vi "Joystick Control.vi"(10 "RobotDriveDevRef":T1={"DevStatus"={"status"=FALSE, "code"=0, "source"=""}, "Motors[]"=[], "Square Inputs"=FALSE, "Max Output"=1.0}) -> ()   [LabVIEW 2019]
uses:
  <vilib>/Rock Robotics/WPI/RobotDrive/WPI_RobotDriveDevRef.ctl
  <vilib>/Rock Robotics/WPI/MotorControl/WPI_MotorControlDeviceRef.ctl
  <vilib>/Rock Robotics/WPI/MotorControl/WPI_MotorControlType.ctl
  <vilib>/Rock Robotics/SystemInterfaces/DIO/FPGA_DIOPWMChannel.ctl
  <vilib>/Rock Robotics/WPI/PWM/WPI_PWMDeadband.ctl
  <vilib>/Rock Robotics/SystemInterfaces/DIO/FPGA_DIOChannel.ctl
  Robot Global Data.vi
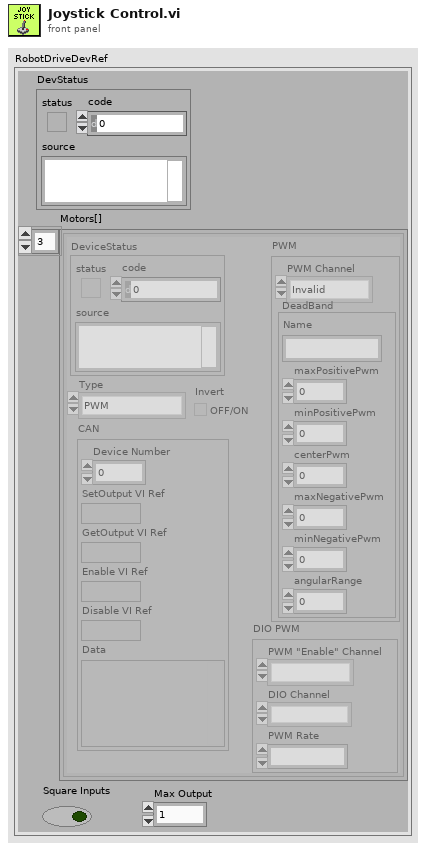
[diagram p1: front panel]
types:
  T1 = typedef "WPI_RobotDriveDevRef.ctl" = cluster{"DevStatus":errorcluster, "Motors[]":T2[], "Square Inputs":bool, "Max Output":dbl}
  T2 = typedef "WPI_MotorControlDeviceRef.ctl" = cluster{"DeviceStatus":errorcluster, "Type":T3, "PWM":cluster{"PWM Channel":T4, "DeadBand":T5}, "CAN":cluster{"Device Number":u8, "SetOutput VI Ref":variant, "GetOutput VI Ref":variant, "Enable VI Ref":variant, "Disable VI Ref":variant, "Data":variant}, "Invert":bool, "DIO PWM":cluster{"PWM \"Enable\" Channel":T4, "DIOChannel":T6, "PWM Rate":dbl}}
  T3 = typedef "WPI_MotorControlType.ctl" = enum16{"PWM", "CAN", "DIO PWM"}
  T4 = typedef "FPGA_DIOPWMChannel.ctl" = enum8{"PWM 0", "PWM 1", "PWM 2", "PWM 3", "PWM 4", "PWM 5", "PWM 6", "PWM 7", "PWM 8", "PWM 9", "PWM MXP 0", "PWM MXP 1", "PWM MXP 2", "PWM MXP 3", "PWM MXP 4", "PWM MXP 5", "PWM MXP 6", "PWM MXP 7", "PWM MXP 8", "PWM MXP 9", "Invalid"}
  T5 = typedef "WPI_PWMDeadband.ctl" = cluster{"Name":string, "maxPositivePwm":i32, "minPositivePwm":i32, "centerPwm":i32, "maxNegativePwm":i32, "minNegativePwm":i32, "angularRange":u16}
  T6 = typedef "FPGA_DIOChannel.ctl" = enum8{"DIO 0", "DIO 1", "DIO 2", "DIO 3", "DIO 4", "DIO 5", "DIO 6", "DIO 7", "DIO 8", "DIO 9", "DIO MXP 0", "DIO MXP 1", "DIO MXP 2", "DIO MXP 3", "DIO MXP 4", "DIO MXP 5", "DIO MXP 6", "DIO MXP 7", "DIO MXP 8", "DIO MXP 9", "DIO MXP 10", "DIO MXP 11", "DIO MXP 12", "DIO MXP 13", "DIO MXP 14", "DIO MXP 15", "SPI Port CS1", "SPI Port CS2", "SPI Port CS3", "SPI Port MISO", "SPI Port MOSI", "Invalid"}
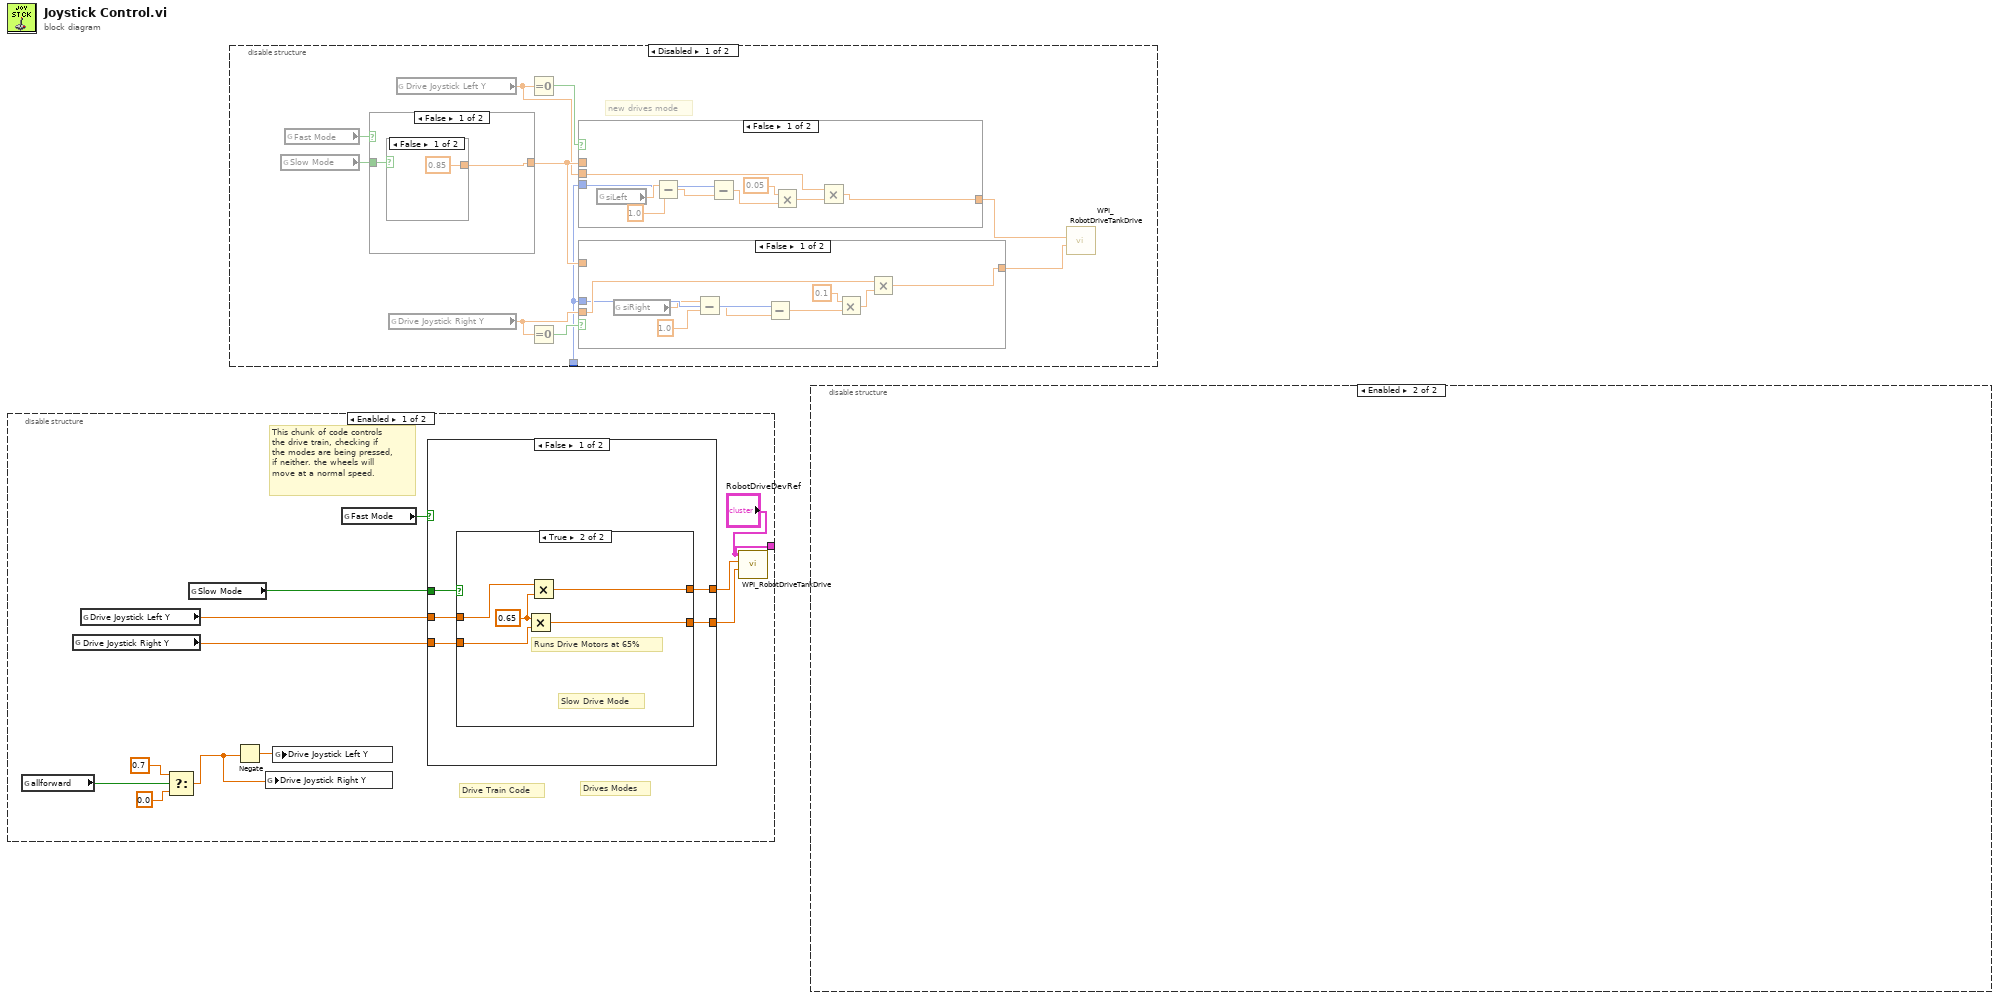
[diagram p0: block diagram]
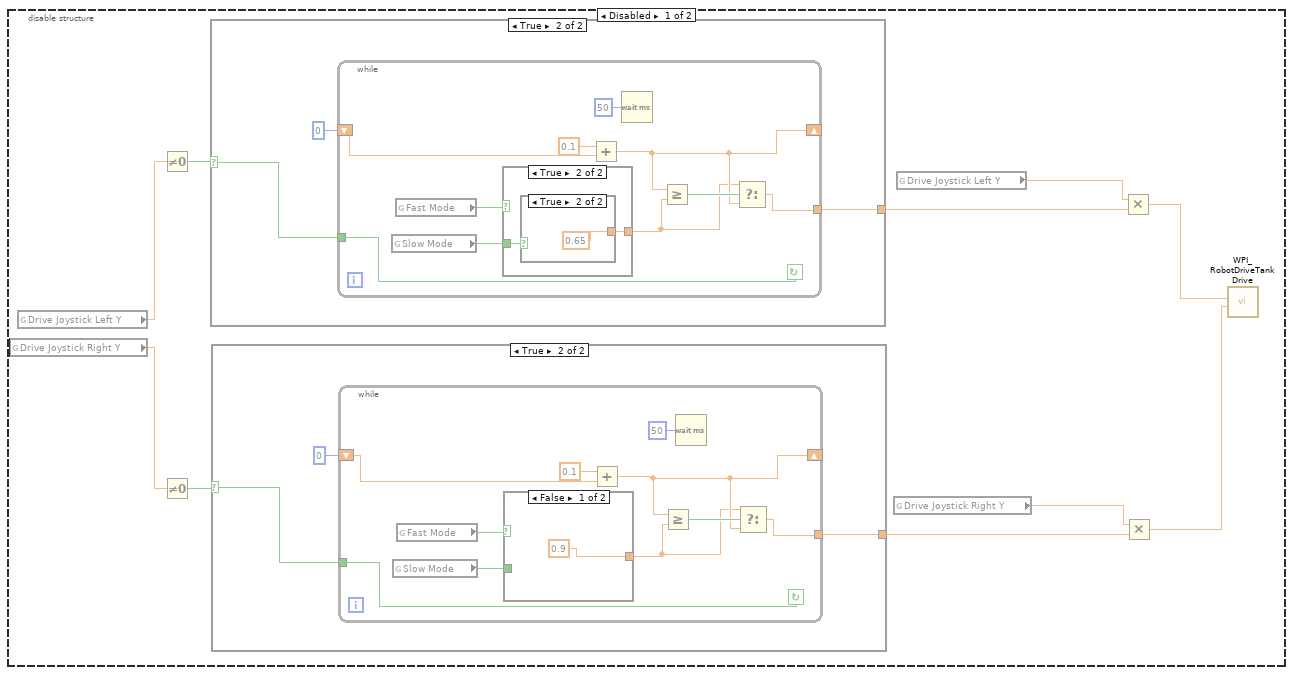
[diagram p2: hidden frame]
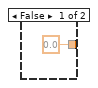
[diagram p3: hidden frame]
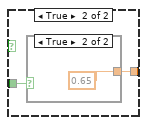
[diagram p4: hidden frame]
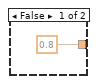
[diagram p5: hidden frame]
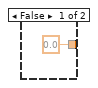
[diagram p6: hidden frame]
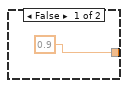
[diagram p7: hidden frame]
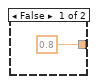
[diagram p8: hidden frame]
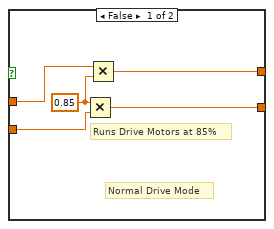
[diagram p9: hidden frame]
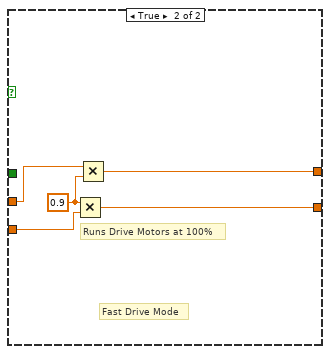
[diagram p10: hidden frame]
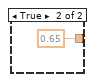
[diagram p12: hidden frame]
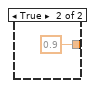
[diagram p13: hidden frame]
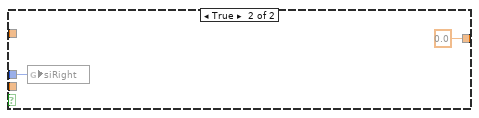
[diagram p14: hidden frame]
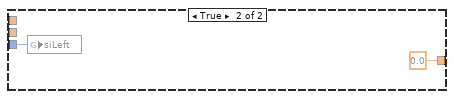
[diagram p15: hidden frame]
diagram:
  n1 = disable-structure shown="Enabled" {
    disable-tunnel: ["RobotDriveDevRef" _] -> _
    frame Enabled {
      # "This chunk of code controls\nthe drive train, checking if \nthe modes are being pressed,\nif neither. the wheels will \nmove at a normal speed."
      # "Drive Train Code"
      # "Drives Modes"
      n2 = global read "Robot Global Data.vi" "allforward"() -> (w5:bool)
      n3 = global read "Robot Global Data.vi" "Drive Joystick Right Y"() -> (w6:dbl)
      n4 = global read "Robot Global Data.vi" "Drive Joystick Left Y"() -> (w7:dbl)
      n5 = Select(t=0.7, s=w5, f=0.0) -> (s? t:f=w1:dbl)
      n6 = global read "Robot Global Data.vi" "Slow Mode"() -> (w12:bool)
      n7 = Negate(x=w1) -> (-x=w2:dbl)
      n8 = global write "Robot Global Data.vi" "Drive Joystick Right Y"(w1) -> ()
      n9 = global write "Robot Global Data.vi" "Drive Joystick Left Y"(w2) -> ()
      n10 = global read "Robot Global Data.vi" "Fast Mode"() -> (w9:bool)
      n11 = case shown="False" w9 {
        tunnel: w7 -> [w16 w32]
        tunnel: w6 -> [w15 w31]
        tunnel: [w14 w29] -> w10
        tunnel: [w13 w28] -> w11
        tunnel: w12 -> [w17 _]
        frame False {
          n12 = case shown="True" w17 {
            tunnel: w16 -> [w21 w26]
            tunnel: w15 -> [w20 w25]
            tunnel: [w19 w24] -> w14
            tunnel: [w18 w23] -> w13
            frame False {
              w22 = 0.85
              # "Normal Drive Mode"
              # "Runs Drive Motors at 85%"
              n13 = Multiply(x=w22, y=w20) -> (x*y=w18:dbl)
              n14 = Multiply(x=w21, y=w22) -> (x*y=w19:dbl)
            }
            frame True {
              w27 = 0.65
              # "Slow Drive Mode"
              # "Runs Drive Motors at 65%"
              n15 = Multiply(x=w27, y=w25) -> (x*y=w23:dbl)
              n16 = Multiply(x=w26, y=w27) -> (x*y=w24:dbl)
            }
          }
        }
        frame True {
          w30 = 0.9
          # "Runs Drive Motors at 100%"
          # "Fast Drive Mode"
          n17 = Multiply(x=w30, y=w31) -> (x*y=w28:dbl)
          n18 = Multiply(x=w32, y=w30) -> (x*y=w29:dbl)
        }
      }
      n19 = call <vilib>:"WPI_RobotDriveTankDrive.vi"("Right axis value"=w11, "Left axis value"=w10, "RobotDriveDevRef"="RobotDriveDevRef") -> ()  [unwired: 6 in, 3 out]
    }
    frame Disabled {
    }
  }
  n20 = disable-structure shown="Disabled" {
    disable-tunnel: _ -> [w33 _]
    frame Disabled {
      # "new drives mode"
      n21 = global read "Robot Global Data.vi" "Slow Mode"() -> (w41:bool)
      n22 = global read "Robot Global Data.vi" "Fast Mode"() -> (w40:bool)
      n23 = case shown="False" w40 {
        tunnel: [w44 0.9] -> w42
        tunnel: w41 -> [w43 _]
        frame False {
          n24 = case shown="False" w43 {
            tunnel: [0.85 0.65] -> w44
            frame False {
            }
            frame True {
            }
          }
        }
        frame True {
        }
      }
      n25 = global read "Robot Global Data.vi" "Drive Joystick Right Y"() -> (w39:dbl)
      n26 = global read "Robot Global Data.vi" "Drive Joystick Left Y"() -> (w38:dbl)
      n27 = Equal To 0?(x=w38) -> (x = 0?=w34:bool)
      n28 = Equal To 0?(x=w39) -> (x = 0?=w36:bool)
      n29 = case shown="False" w34 {
        tunnel: w33 -> [w61 w69]
        tunnel: [w59 0.0 ("x")] -> w35
        tunnel: w38 -> [w64 _]
        tunnel: w42 -> [_ _]
        frame False {
          n30 = global read "Robot Global Data.vi" "siLeft"() -> (w63:dbl)
          n31 = Subtract(x=w63, y=1.0) -> (x-y=w60:dbl)
          n32 = Subtract(x=w61, y=w60) -> (x-y=w67:dbl)
          n33 = Multiply(x=0.05, y=w67) -> (x*y=w65:dbl)
          n34 = Multiply(x=w64, y=w65) -> (x*y=w59:dbl)
        }
        frame True {
          n35 = global write "Robot Global Data.vi" "siLeft"(w69) -> ()
        }
      }
      n36 = case shown="False" w36 {
        tunnel: [w48 0.0 ("x")] -> w37
        tunnel: w33 -> [w52 w57]
        tunnel: w39 -> [w53 _]
        tunnel: w42 -> [_ _]
        frame False {
          n37 = global read "Robot Global Data.vi" "siRight"() -> (w51:dbl)
          n38 = Subtract(x=w51, y=1.0) -> (x-y=w50:dbl)
          n39 = Subtract(x=w52, y=w50) -> (x-y=w56:dbl)
          n40 = Multiply(x=0.1, y=w56) -> (x*y=w54:dbl)
          n41 = Multiply(x=w53, y=w54) -> (x*y=w48:dbl)
        }
        frame True {
          n42 = global write "Robot Global Data.vi" "siRight"(w57) -> ()
        }
      }
      n43 = call <vilib>:"WPI_RobotDriveTankDrive.vi"("Right axis value"=w37, "Left axis value"=w35) -> ()  [unwired: 7 in, 3 out]
    }
    frame Enabled {
    }
  }
  n44 = disable-structure shown="Enabled" {
    frame Disabled {
      n45 = global read "Robot Global Data.vi" "Drive Joystick Right Y"() -> (w70:dbl)
      n46 = global read "Robot Global Data.vi" "Drive Joystick Left Y"() -> (w71:dbl)
      n47 = Not Equal To 0?(x=w71) -> (x != 0?=w79:bool)
      n48 = Not Equal To 0?(x=w70) -> (x != 0?=w75:bool)
      n49 = case shown="True" w79 {
        selector: w79 -> [_ w100]
        tunnel: [0.0 w101] -> w78
        frame False {
        }
        frame True {
          n50 = while {
            shift-right: [w107] -> _
            shift-left: 0 -> [w103]
            tunnel: w100 -> [w111]
            tunnel: [w105] -> w101
            stop <- w111 continue-if-true
            n51 = global read "Robot Global Data.vi" "Slow Mode"() -> (w108:bool)
            n52 = global read "Robot Global Data.vi" "Fast Mode"() -> (w109:bool)
            n53 = case shown="True" w109 {
              tunnel: w108 -> [_ w115]
              tunnel: [0.9 w114] -> w106
              frame False {
              }
              frame True {
                n54 = case shown="True" w115 {
                  tunnel: [0.8 0.65] -> w114
                  frame False {
                  }
                  frame True {
                  }
                }
              }
            }
            n55 = Add(x=0.1, y=w103) -> (x+y=w107:dbl)
            n56 = Wait (ms)(milliseconds to wait=u32 50) -> ()  [unwired: 1 out]
            n57 = Greater Or Equal?(x=w107, y=w106) -> (x >= y?=w110:bool)
            n58 = Select(t=w106, s=w110, f=w107) -> (s? t:f=w105:dbl)
          }
        }
      }
      n59 = case shown="True" w75 {
        selector: w75 -> [_ w82]
        tunnel: [0.0 w81] -> w76
        frame False {
        }
        frame True {
          n60 = while {
            shift-right: [w87] -> _
            shift-left: 0 -> [w93]
            tunnel: w82 -> [w91]
            tunnel: [w85] -> w81
            stop <- w91 continue-if-true
            n61 = global read "Robot Global Data.vi" "Slow Mode"() -> (w88:bool)
            n62 = global read "Robot Global Data.vi" "Fast Mode"() -> (w89:bool)
            n63 = case shown="False" w89 {
              tunnel: w88 -> [_ w96]
              tunnel: [0.9 w95] -> w86
              frame False {
              }
              frame True {
                n64 = case shown="True" w96 {
                  tunnel: [0.8 0.65] -> w95
                  frame False {
                  }
                  frame True {
                  }
                }
              }
            }
            n65 = Add(x=0.1, y=w93) -> (x+y=w87:dbl)
            n66 = Greater Or Equal?(x=w87, y=w86) -> (x >= y?=w90:bool)
            n67 = Wait (ms)(milliseconds to wait=u32 50) -> ()  [unwired: 1 out]
            n68 = Select(t=w86, s=w90, f=w87) -> (s? t:f=w85:dbl)
          }
        }
      }
      n69 = global read "Robot Global Data.vi" "Drive Joystick Right Y"() -> (w72:dbl)
      n70 = global read "Robot Global Data.vi" "Drive Joystick Left Y"() -> (w73:dbl)
      n71 = Multiply(x=w73, y=w78) -> (x*y=w77:dbl)
      n72 = Multiply(x=w72, y=w76) -> (x*y=w74:dbl)
      n73 = call <vilib>:"WPI_RobotDriveTankDrive.vi"("Right axis value"=w74, "Left axis value"=w77) -> ()  [unwired: 7 in, 3 out]
    }
    frame Enabled {
    }
  }
